vi "Static DAQ prog.vi"(3 "device":i16=1, 4 "Voltage Array":dbl[][](array[numeric]) format="%.2f") -> (1 "task out":refnum<k21>)   [LabVIEW 2017]
doc: "This vi programs the Static DAQ. The inputs are an array of voltages (in volts), with one collumn per channel, and a device number for the DAQ card. (The device number can be found in NI's Measurement&Automation Explorer in Configurations: Devices and Interfaces:Traditional NI-DAQ devices)."
uses:
  <vilib>/Utility/error.llb/DialogType.ctl
  <vilib>/DAQmx/write.llb/DAQmx Write (Analog 2D DBL NChan NSamp).vi
  <vilib>/DAQmx/create/channels.llb/DAQmx Create Channel (AO-Voltage-Basic).vi
  <vilib>/DAQmx/configure/timing.llb/DAQmx Timing (Sample Clock).vi
  <vilib>/DAQmx/miscellaneous.llb/DAQmx Fill In Error Info.vi
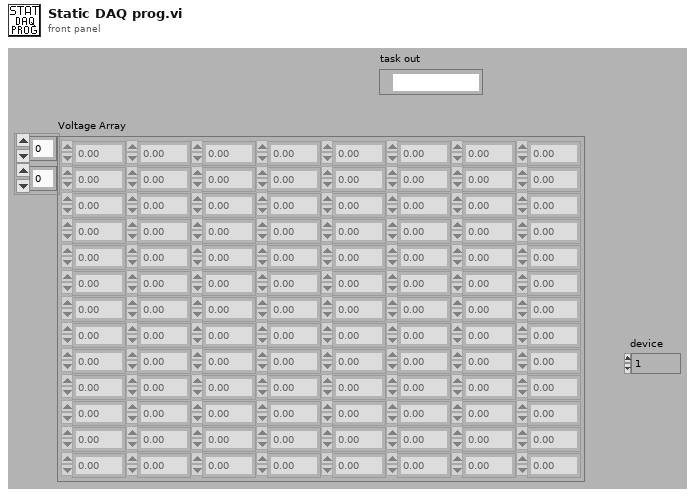
[diagram p1: front panel]
types:
  T1 = typedef "DialogType.ctl" = u16
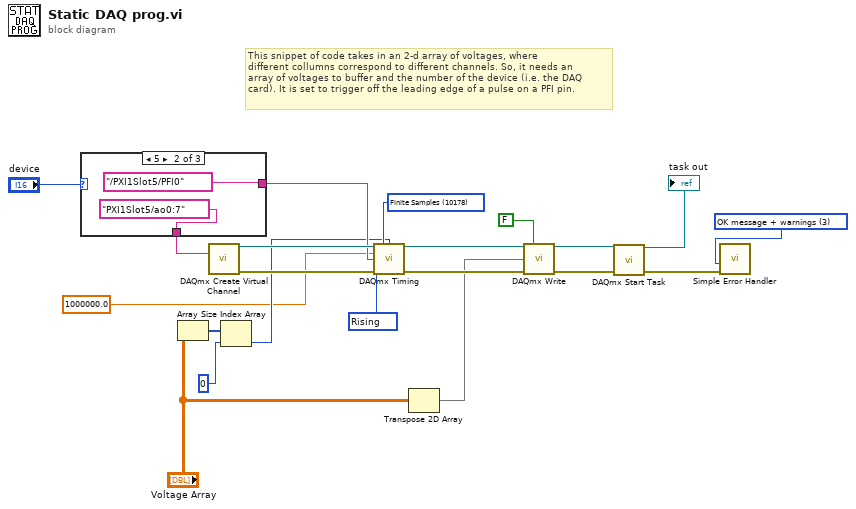
[diagram p0: block diagram]
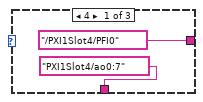
[diagram p2: hidden frame]
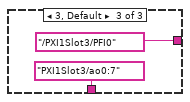
[diagram p3: hidden frame]
diagram:
  w2 = T1 3 items=["no dialog", "OK message", "continue or stop message", "OK message + warnings", "continue/stop + warnings"] ("type of dialog (OK msg:1)")
  w11 = 10178 items=["Finite Samples"=10178, "Continuous Samples"=10123, "Hardware Timed Single Point"=12522] ("sample mode")
  w17 = 10280 items=["Rising"=10280, "Falling"=10171] ("active edge")
  # "This snippet of code takes in an 2-d array of voltages, where\ndifferent collumns correspond to different channels. So, it needs an\narray of voltages to buffer and the number of the device (i.e. the DAQ\ncard). It is set to trigger off the leading edge of a pulse on a PFI pin."
  n1 = case shown="5" "device" {
    tunnel: [tag "PXI1Slot4/ao0:7" ("physical channels") tag "PXI1Slot5/ao0:7" ("physical channels") tag "PXI1Slot3/ao0:7" ("physical channels")] -> w9
    tunnel: [tag "/PXI1Slot4/PFI0" ("source") tag "/PXI1Slot5/PFI0" ("source") tag "/PXI1Slot3/PFI0" ("source")] -> w8
    frame 4 {
    }
    frame 5 {
    }
    frame 3, Default {
    }
  }
  n2 = Array Size(array="Voltage Array") -> (size(s)=w21:i32[])
  n3 = call-poly <vilib>:"DAQmx Create Virtual Channel.vi"("physical channels"=w9) -> ("task out"=w18:refnum<k21>, "error out"=w19:errorcluster)  [unwired: 13 in]
  n4 = Index Array(array=w21, index=0 ("Index")) -> (element=w7:i32)
  n5 = call-poly <vilib>:"DAQmx Timing.vi"("task/channels in"=w18, "sample mode"=w11, "samples per channel"=w7, "rate"=1000000.0, "source"=w8, "active edge"=w17, "error in"=w19) -> ("task out"=w16:refnum<k21>, "error out"=w13:errorcluster)  [unwired: 7 in]
  n6 = Transpose 2D Array(2D array="Voltage Array") -> (transposed array=w3:dbl[][])
  n7 = call-poly <vilib>:"DAQmx Write.vi"("task/channels in"=w16, "auto start"=FALSE, "data"=w3, "error in"=w13) -> ("task out"=w15:refnum<k21>, "error out"=w12:errorcluster)  [unwired: 9 in, 1 out]
  n8 = call <vilib>:"DAQmx Start Task.vi"("task/channels in"=w15, "error in"=w12) -> ("task out"=→"task out":refnum<k21>, "error out"=w1:errorcluster)  [unwired: 12 in]
  n9 = call <vilib>:"Simple Error Handler.vi"("type of dialog (OK msg:1)"=w2, "error in (no error)"=w1) -> ()  [unwired: 3 in, 5 out]
